vi "Get Tag.vi"(8 "Error In":errorcluster, 11 "Animation In":refnum<class "Animation.lvclass">) -> (0 "Error Out":errorcluster, 2 "Tag":string, 3 "Animation Out":refnum<class "Animation.lvclass">)   [LabVIEW 2021, in "Animation.lvclass"]
uses:
  Animation.lvclass
  Animation.lvclass/Animation.ctl
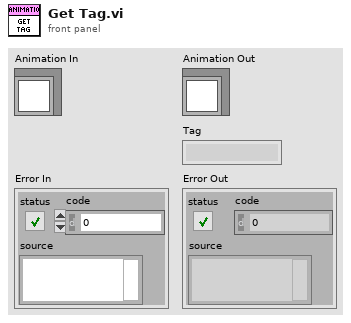
[diagram p1: front panel]
types:
  T1 = typedef "Animation.lvclass/Data.ctl" = cluster{"Tag":string}
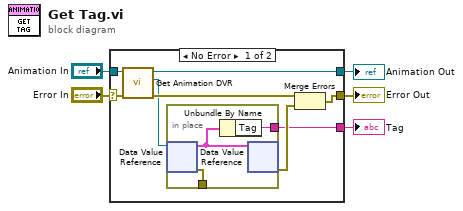
[diagram p0: block diagram]
diagram:
  n1 = case shown="No Error" "Error In" {
    selector: "Error In" -> [w9 w17]
    tunnel: [w11 w17] -> w4
    tunnel: [w8 w18] -> w2
    tunnel: "Animation In" -> [w10 w18]
    tunnel: [w12 _] -> w1
    frame No Error {
      n2 = call "Get Animation DVR.vi"("Error In"=w9, "Animation In"=w10) -> ("Error Out"=w7:errorcluster, "DVR"=w6:refnum<data-value>, "Animation Out"=w8:refnum<class "Animation.lvclass">)  [unwired: 7 in]
      n3 = in-place {
        in-place-border: [w14] -> w12
        in-place-border: [w16] -> _
        n4 = in-place-dvr #1(w6) -> (w15:T1, w16:errorcluster)
        n5 = Unbundle By Name(w15) -> ("Tag"=w14:string)
        n6 = in-place-dvr #1(w15) -> (w13:errorcluster)  [unwired: 1 out]
      }
      n7 = Merge Errors(w7, w13) -> (w11:errorcluster)
    }
    frame Error {
    }
  }
  "Animation Out" <- w2
  "Error Out" <- w4
  "Tag" <- w1
